vi "Find.vi"(8 "Error In":errorcluster, 10 "Key":string, 11 "Context In":refnum<class "Context.lvclass">) -> (0 "Error Out":errorcluster, 1 "Found?":bool, 2 "Datum":refnum<class "Datum.lvclass">, 3 "Context Out":refnum<class "Context.lvclass">)   [LabVIEW 2018, in "Toolkit.lvlib" / "Context.lvclass"]
doc: "Finds a value associated with the key within the context."
uses:
  Context.lvclass
  Data/Datum/Datum.lvclass
  Context.lvclass/Context.ctl
  Data/Null/Null.lvclass
  D:/Users/cfield/Code/Field R&D Services/Labstache/src/Toolkit/Data/Datum/Datum.lvclass
  Data/Map/Map.lvclass
  Data/Pair/Pair.lvclass
  Data/Pair/Pair.lvclass/Pair.ctl
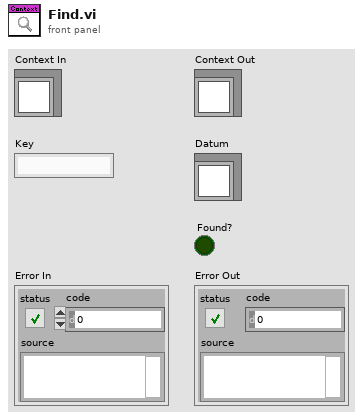
[diagram p1: front panel]
types:
  T1 = typedef "Toolkit.lvlib/Data.lvlib/Types.ctl" = enum16{"Array", "Boolean", "Function", "Map", "Null", "Pair", "Path", "String", "Unknown"}
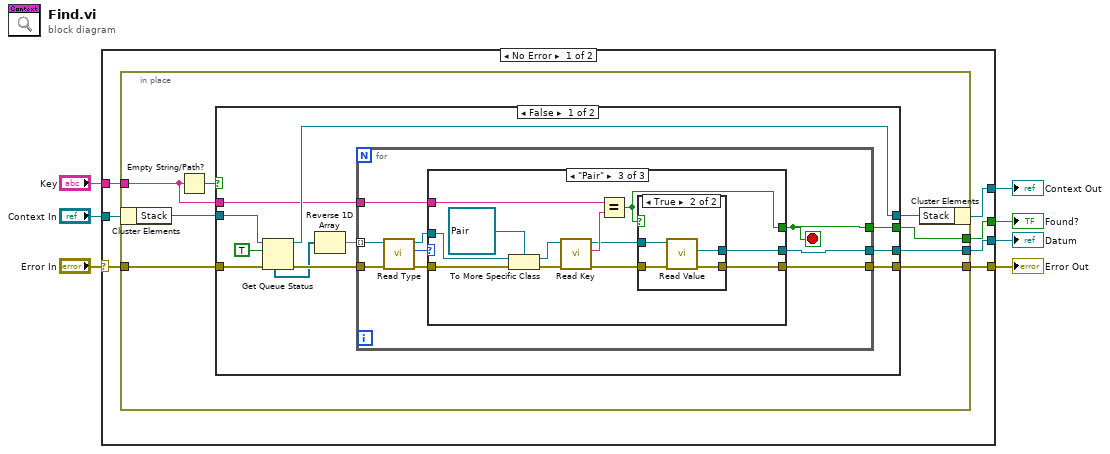
[diagram p0: block diagram]
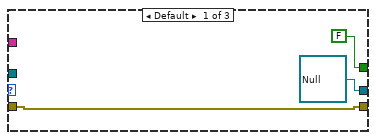
[diagram p2: hidden frame]
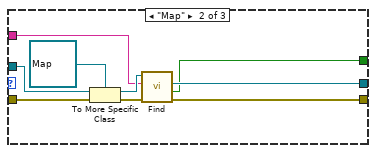
[diagram p3: hidden frame]
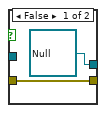
[diagram p4: hidden frame]
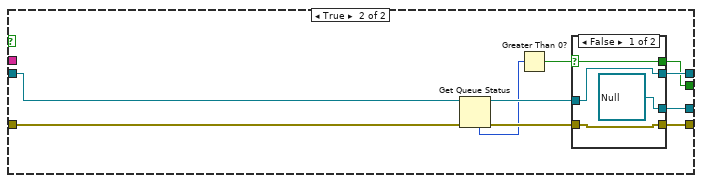
[diagram p5: hidden frame]
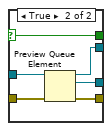
[diagram p6: hidden frame]
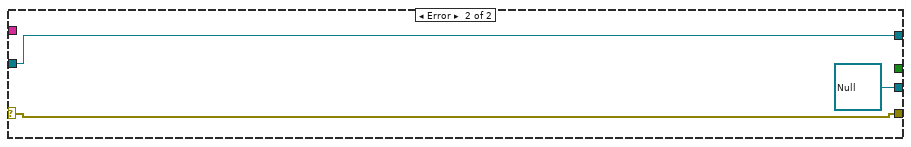
[diagram p7: hidden frame]
diagram:
  n1 = case shown="No Error" "Error In" {
    selector: "Error In" -> [w11 w94]
    tunnel: [w14 refnum<class "Null.lvclass"> refnum ("Toolkit.lvlib:Data.lvlib:Null.lvclass")] -> w7
    tunnel: [w13 w94] -> w6
    tunnel: [w12 _] -> w5
    tunnel: "Context In" -> [w10 w95]
    tunnel: [w9 w95] -> w2
    tunnel: "Key" -> [w8 _]
    frame No Error {
      n2 = in-place {
        in-place-border: [w22] -> w14
        in-place-border: [w21] -> w13
        in-place-border: [w20] -> w12
        in-place-border: w11 -> [w19]
        in-place-border: w8 -> [w16]
        n3 = in-place-cluster #1(w10) -> ("Stack"=w18:refnum<queue>)
        n4 = Empty String/Path?(string/path=w16) -> (empty?=w15:bool)
        n5 = case shown="False" w15 {
          tunnel: [w33 w81] -> w22
          tunnel: [w32 w73] -> w21
          tunnel: [w27 w74] -> w20
          tunnel: w19 -> [w26 w77]
          tunnel: w18 -> [w25 w80]
          tunnel: [w24 w82] -> w17
          tunnel: w16 -> [w23 _]
          frame False {
            n6 = Get Queue Status(queue=w25, return elements? (F)=TRUE, error in (no error)=w26) -> (queue out=w24:refnum<queue>, error out=w31:errorcluster, elements=w29:refnum<class "Datum.lvclass">[])  [unwired: 5 out]
            n7 = Reverse 1D Array(array=w29) -> (reversed array=w30:refnum<class "Datum.lvclass">[])
            n8 = for {
              tunnel: w30 -> [w38] mode=indexing
              tunnel: w23 -> [w42]
              tunnel: w31 -> [w36]
              tunnel: [w41] -> w32
              tunnel: [w40] -> w33
              tunnel: [w39] -> w27
              stop <- w39 stop-if-true
              n9 = call-dynamic "Read Type.vi"("Error In"=w36, "Datum In"=w38) -> ("Error Out"=w35:errorcluster, "Type"=w34:T1, "Datum Out"=w37:refnum<class "Datum.lvclass">)  [unwired: 7 in]
              n10 = case shown="\"Pair\"" w34 {
                tunnel: w35 -> [w44 w54 w66]
                tunnel: w37 -> [_ w53 w65]
                tunnel: w42 -> [_ w49 w60]
                tunnel: [w44 w48 w57] -> w41
                tunnel: [FALSE ("Found?") w46 w59] -> w39
                tunnel: [refnum<class "Null.lvclass"> refnum ("Toolkit.lvlib:Data.lvlib:Null.lvclass") w47 w55] -> w40
                frame Default {
                }
                frame "Map" {
                  n11 = To More Specific Class(target class=refnum<class "Map.lvclass"> refnum ("Toolkit.lvlib:Data.lvlib:Map.lvclass"), reference=w53, error in=w54) -> (specific class reference=w50:refnum<class "Map.lvclass">, error out=w51:errorcluster)
                  n12 = call "Find.vi"("Error In"=w51, "Key"=w49, "Map In"=w50) -> ("Error Out"=w48:errorcluster, "Found?"=w46:bool, "Value"=w47:refnum<class "Datum.lvclass">)  [unwired: 5 in, 1 out]
                }
                frame "Pair" {
                  n13 = To More Specific Class(target class=refnum<class "Pair.lvclass"> refnum ("Toolkit.lvlib:Data.lvlib:Pair.lvclass"), reference=w65, error in=w66) -> (specific class reference=w63:refnum<class "Pair.lvclass">, error out=w62:errorcluster)
                  n14 = call "Read Key.vi"("Error In"=w62, "Pair In"=w63) -> ("Error Out"=w58:errorcluster, "Key"=w61:string, "Pair Out"=w56:refnum<class "Pair.lvclass">)  [unwired: 7 in]
                  n15 = Equal?(x=w60, y=w61) -> (x = y?=w59:bool)
                  n16 = case shown="True" w59 {
                    tunnel: w58 -> [w68 w72]
                    tunnel: [w68 w71] -> w57
                    tunnel: w56 -> [_ w70]
                    tunnel: [refnum<class "Null.lvclass"> refnum ("Toolkit.lvlib:Data.lvlib:Null.lvclass") w69] -> w55
                    frame False {
                    }
                    frame True {
                      n17 = call "Read Value.vi"("Error In"=w72, "Pair In"=w70) -> ("Error Out"=w71:errorcluster, "Value"=w69:refnum<class "Datum.lvclass">)  [unwired: 7 in, 1 out]
                    }
                  }
                }
              }
            }
          }
          frame True {
            n18 = Get Queue Status(queue=w80, error in (no error)=w77) -> (queue out=w79:refnum<queue>, error out=w78:errorcluster, # elements in queue=w76:i32)  [unwired: 1 in, 5 out]
            n19 = Greater Than 0?(x=w76) -> (x > 0?=w75:bool)
            n20 = case shown="False" w75 {
              selector: w75 -> [w85 w87]
              tunnel: [w86 w92] -> w82
              tunnel: [refnum<class "Null.lvclass"> refnum ("Toolkit.lvlib:Data.lvlib:Null.lvclass") w91] -> w81
              tunnel: w79 -> [w86 w90]
              tunnel: w78 -> [w84 w89]
              tunnel: [w85 w87] -> w74
              tunnel: [w84 w88] -> w73
              frame False {
              }
              frame True {
                n21 = Preview Queue Element(queue=w90, error in (no error)=w89) -> (queue out=w92:refnum<queue>, element=w91:refnum<class "Datum.lvclass">, error out=w88:errorcluster)  [unwired: 1 in, 1 out]
              }
            }
          }
        }
        n22 = in-place-cluster #1("Stack"=w17) -> (w9:refnum<class "Context.lvclass">)
      }
    }
    frame Error {
    }
  }
  "Datum" <- w7
  "Error Out" <- w6
  "Found?" <- w5
  "Context Out" <- w2
